vi "Chamber_Unfill.vi"(8 "error in (no error)":errorcluster, 11 "Data Cluster in":T1 {"Display"."Coffee" scale=0.0..80.0; "Display"."Chamber" scale=0.0..80.0; "Controls"."Type" scale=0.0..2.0; "Simulators"."Milk Level" min=0.0 max=100.0 step=10.0 scale=0.0..100.0 scale format="%#_3g"; "Simulators"."Bean Level" min=0.0 max=100.0 step=10.0 scale=0.0..100.0 scale format="%#_3g"; "Simulators"."Water Level" min=0.0 max=100.0 step=10.0 scale=0.0..100.0 scale format="%#_3g"}) -> (0 "error out":errorcluster, 3 "Data Cluster out":T1 {"Display"."Coffee" scale=0.0..80.0; "Display"."Chamber" scale=0.0..80.0; "Controls"."Type" scale=0.0..2.0; "Simulators"."Milk Level" min=0.0 max=100.0 step=10.0 scale=0.0..100.0 scale format="%#_3g"; "Simulators"."Bean Level" min=0.0 max=100.0 step=10.0 scale=0.0..100.0 scale format="%#_3g"; "Simulators"."Water Level" min=0.0 max=100.0 step=10.0 scale=0.0..100.0 scale format="%#_3g"})   [LabVIEW 2026]
uses:
  controls/UI Data.ctl
  controls/Simulators.ctl
  controls/Controls.ctl
  controls/Type_Enum.ctl
  controls/Display.ctl
  controls/System_Status.ctl
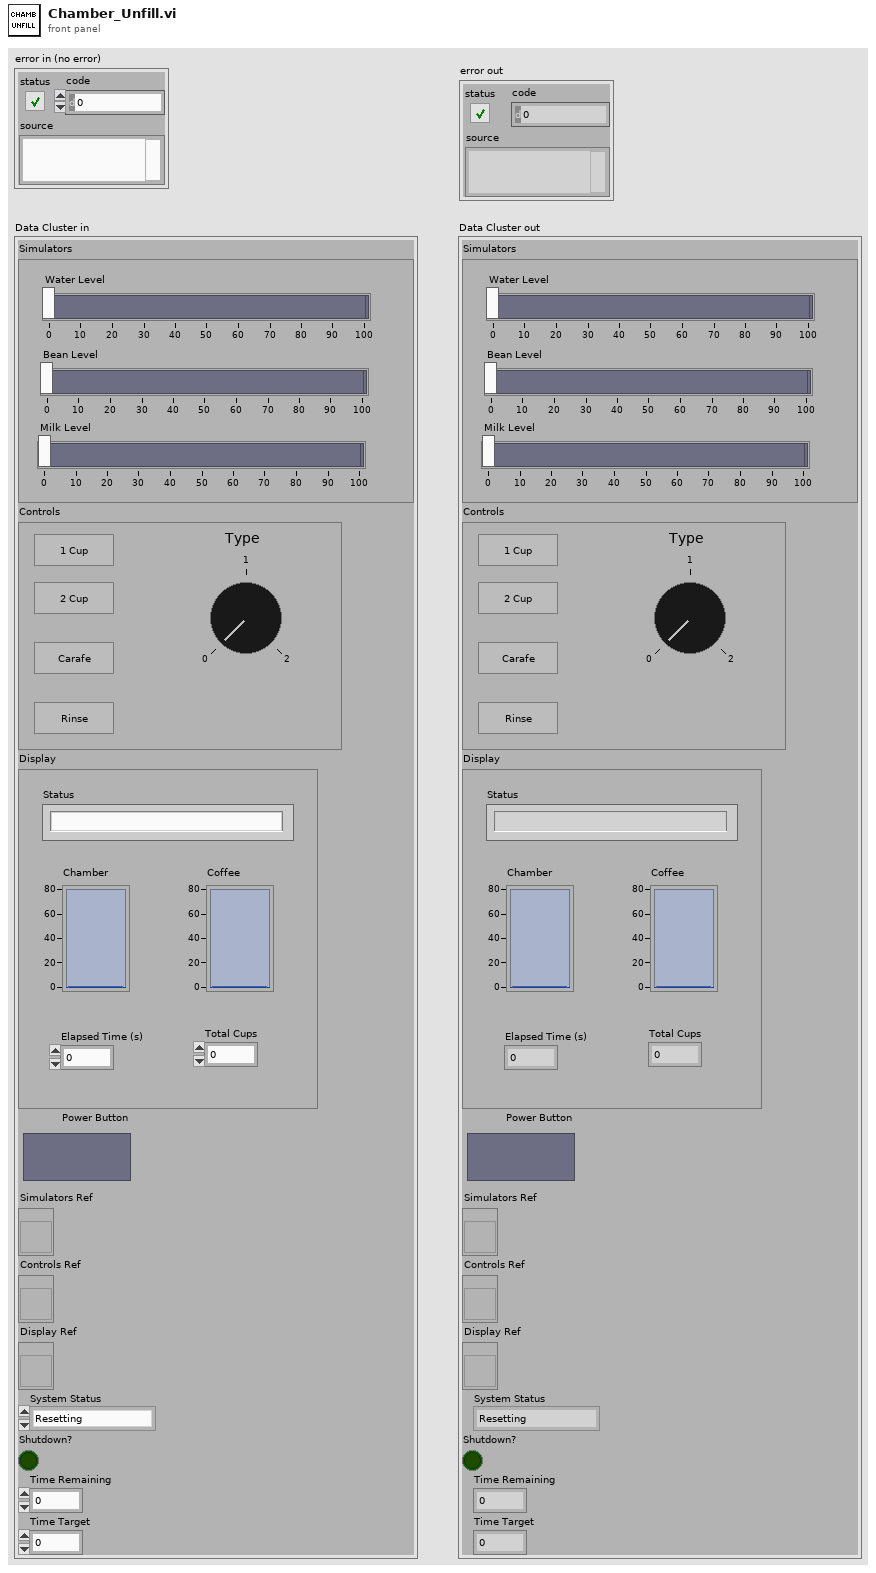
[diagram p1: front panel]
types:
  T1 = typedef "UI Data.ctl" = cluster{"Simulators":T2, "Controls":T3, "Display":T5, "Power Button":bool, "Simulators Ref":refnum<vi>, "Controls Ref":refnum<vi>, "Display Ref":refnum<vi>, "System Status":T6, "Shutdown?":bool, "Time Remaining":dbl, "Time Target":dbl}
  T2 = typedef "Simulators.ctl" = cluster{"Water Level":dbl, "Bean Level":dbl, "Milk Level":dbl}
  T3 = typedef "Controls.ctl" = cluster{"1 Cup":bool, "2 Cup":bool, "Carafe":bool, "Rinse":bool, "Type":T4}
  T4 = typedef "Type_Enum.ctl" = i16
  T5 = typedef "Display.ctl" = cluster{"Status":string, "Chamber":dbl, "Coffee":dbl, "Elapsed Time (s)":dbl, "Total Cups":dbl}
  T6 = typedef "System_Status.ctl" = enum16{"Resetting", "Heating Up", "Rinsing", "Threshold Check", "Ready for Brewing", "Grinding", "Brewing", "Dispensing", "Stepping", "Fulfilling", "Shutting Down"}
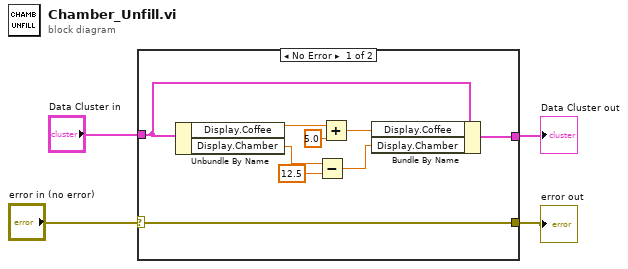
[diagram p0: block diagram]
diagram:
  n1 = case shown="No Error" "error in (no error)" {
    selector: "error in (no error)" -> [w9 w15]
    tunnel: [w13 w14] -> w4
    tunnel: "Data Cluster in" -> [w12 w14]
    tunnel: [w9 w15] -> w1
    frame No Error {
      n2 = Unbundle By Name(w12) -> ("Display.Coffee"=w10:dbl, "Display.Chamber"=w6:dbl)
      n3 = Subtract(x=w6, y=12.5) -> (x-y=w7:dbl)
      n4 = Add(x=w10, y=5.0) -> (x+y=w11:dbl)
      n5 = Bundle By Name(cluster=w12, "Display.Coffee"=w11, "Display.Chamber"=w7) -> (w13:T1)
    }
    frame Error {
    }
  }
  "Data Cluster out" <- w4
  "error out" <- w1
